vi "Record Zernike Sequence.vi"(7 "Zernike Optimize Settings":T1={"ZO Settings"={"Acquisition Settings"={"Save?"=FALSE, "DCIMG Path"=path "", "Filename"="", "Total Frames"=0, "Sender"=enum."UI"}, "Shift Amplitude"=0.0, "Initial Zernike Vector"=[]}, "Zernike Size"=15, "Points per order"=15, "Zernike State"=enum."Idle", "Zernike Vectors"=[], "Total Frames"=15, "Current Frame"=15}, 8 "error in":errorcluster, 9 "Camera":refnum<queue>, 10 "DM":refnum<queue>, 11 "Z_0":dbl[](array[numeric])) -> (0 "error out":errorcluster)   [LabVIEW 2015, in "Automation.lvlib"]
uses:
  Automation.lvlib
  support/Message Queue/Message Cluster.ctl
  ZO State.ctl
  ZO Settings.ctl
  Camera/Acquisition Settings.ctl
  support/Message Queue/Message Queue.lvlib
  Camera/Camera.lvlib
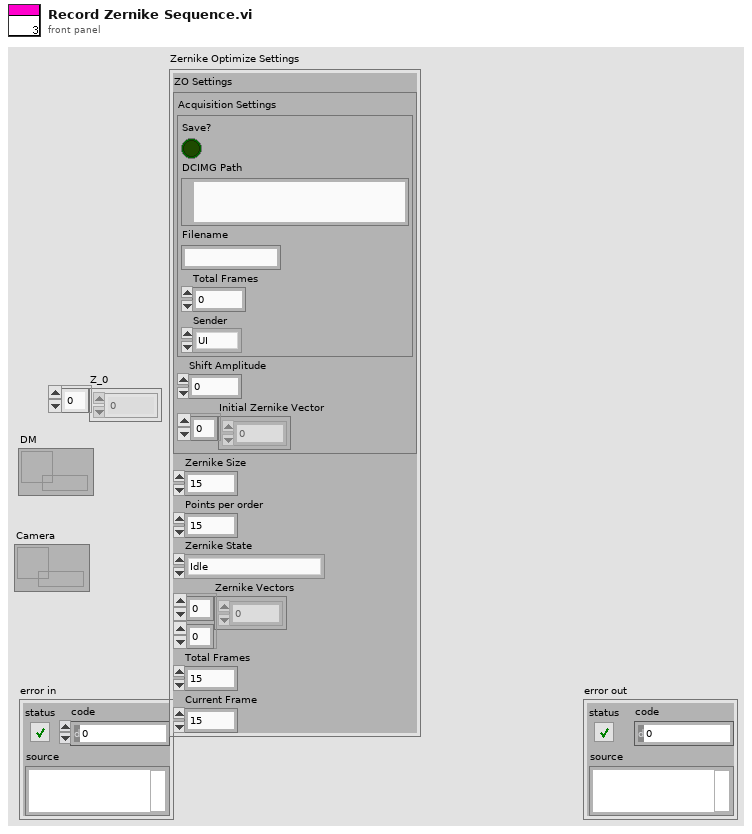
[diagram p1: front panel]
types:
  T1 = typedef "Automation.lvlib/ZO State.ctl" = cluster{"ZO Settings":T2, "Zernike Size":i32, "Points per order":i32, "Zernike State":enum16{"Idle", "Waiting for Camera Init.", "Wait for camera frame", "Ready for new mirror config"}, "Zernike Vectors":dbl[][], "Total Frames":i32, "Current Frame":i32}
  T2 = typedef "Automation.lvlib/ZO Settings.ctl" = cluster{"Acquisition Settings":T3, "Shift Amplitude":dbl, "Initial Zernike Vector":dbl[]}
  T3 = typedef "Camera.lvlib/Acquisition Settings.ctl" = cluster{"Save?":bool, "DCIMG Path":path, "Filename":string, "Total Frames":i32, "Sender":enum16{"UI", "Automation"}}
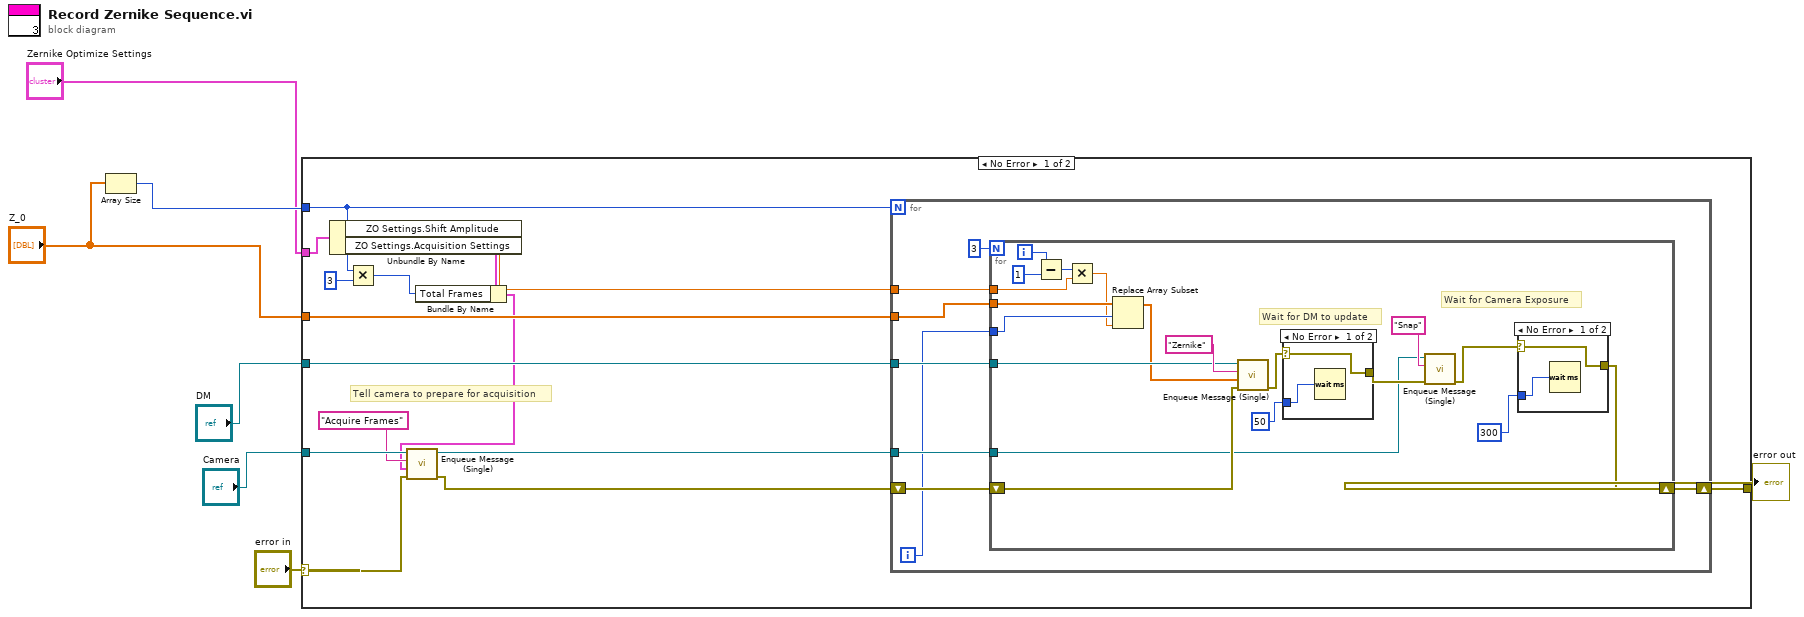
[diagram p0: block diagram]
diagram:
  n1 = Array Size(array="Z_0") -> (size(s)=w2:i32)
  n2 = case shown="No Error" "error in" {
    selector: "error in" -> [w18 w56]
    tunnel: [w15 w56] -> w6
    tunnel: w2 -> [w11 _]
    tunnel: "Z_0" -> [w22 _]
    tunnel: "DM" -> [w21 _]
    tunnel: "Camera" -> [w20 _]
    tunnel: "Zernike Optimize Settings" -> [w14 _]
    frame No Error {
      # "Tell camera to prepare for acquisition"
      n3 = Unbundle By Name(w14) -> ("ZO Settings.Shift Amplitude"=w13:dbl, "ZO Settings.Acquisition Settings"=w12:T3)
      n4 = Multiply(x=w11, y=3) -> (x*y=w9:i32)
      n5 = Bundle By Name(cluster=w12, "Total Frames"=w9) -> (w8:T3)
      n6 = call "Enqueue Message (Single).vi"("error in (no error)"=w18, "Message Data"=w8, "Message"="Acquire Frames", "Message Queue"=w20) -> ("error out"=w17:errorcluster, "dup Message Queue"=w16:refnum<queue>)  [unwired: 6 in]
      n7 = for {
        N: w11 -> [_]
        tunnel: w22 -> [w29]
        tunnel: w13 -> [w28]
        tunnel: w21 -> [w27]
        tunnel: w16 -> [w25]
        shift-right: [w24] -> w15
        shift-left: w17 -> [w26]
        i -> [w23]
        n8 = for {
          N: 3 -> [_]
          tunnel: w29 -> [w49]
          tunnel: w23 -> [w48]
          tunnel: w28 -> [w45]
          tunnel: w27 -> [w42]
          tunnel: w25 -> [w35]
          shift-right: [w33] -> w24
          shift-left: w26 -> [w40]
          i -> [w31]
          # "Wait for Camera Exposure"
          # "Wait for DM to update"
          n9 = Subtract(x=w31, y=1) -> (x-y=w46:i32)
          n10 = Multiply(x=w46, y=w45) -> (x*y=w44:dbl)
          n11 = Replace Array Subset(array=w49, new element=w44, index=w48) -> (w41:dbl[])
          n12 = call "Enqueue Message (Single).vi"("error in (no error)"=w40, "Message Data"=w41, "Message"="Zernike", "Message Queue"=w42) -> ("error out"=w39:errorcluster)  [unwired: 6 in, 1 out]
          n13 = case shown="No Error" w39 {
            selector: w39 -> [w53 w55]
            tunnel: u32 50 ("milliseconds to wait") -> [w54 _]
            tunnel: [w53 w55] -> w37
            frame No Error {
              n14 = Wait (ms)(milliseconds to wait=w54) -> ()  [unwired: 1 out]
            }
            frame Error {
            }
          }
          n15 = call "Enqueue Message (Single).vi"("error in (no error)"=w37, "Message"="Snap", "Message Queue"=w35) -> ("error out"=w34:errorcluster)  [unwired: 7 in, 1 out]
          n16 = case shown="No Error" w34 {
            selector: w34 -> [w50 w52]
            tunnel: u32 300 ("milliseconds to wait") -> [w51 _]
            tunnel: [w50 w52] -> w33
            frame No Error {
              n17 = Wait (ms)(milliseconds to wait=w51) -> ()  [unwired: 1 out]
            }
            frame Error {
            }
          }
        }
      }
    }
    frame Error {
    }
  }
  "error out" <- w6
